vi "Configure Trigger.vi"   [LabVIEW 2012, in "Tektronix TDS 200 1000 2000 Series.lvlib"]
doc: "Allows user to select Edge, Pulse, or Video triggering.\n\n<B>Edge</B> (default) - Triggers the oscilloscope on the rising or falling edge of the input signal when it crosses the trigger level (threshold).\n\n<B>Video</B> - Displays NTSC or PAL/SECAM standard composite video waveforms; you trigger on fields or lines of video signals. \n\n<B>Pulse</B> - Triggers on aberrant pulses."
uses:
  <instrlib>/Tektronix TDS 200 1000 2000 Series/Tektronix TDS 200 1000 2000 Series.lvlib
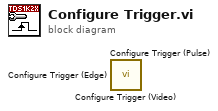
[diagram p0: block diagram]
diagram:
  n1 = call <instrlib>:"Configure Trigger (Video).vi"() -> ()  [unwired: 14 in, 2 out]
  n2 = call <instrlib>:"Configure Trigger (Pulse).vi"() -> ()  [unwired: 14 in, 2 out]
  n3 = call <instrlib>:"Configure Trigger (Edge).vi"() -> ()  [unwired: 14 in, 2 out]
